vi "Asylum_Driver_GetXYSetPoints.vi"(8 "error in (no error)":errorcluster, 11 "Application":refnum<k7>) -> (0 "error out":errorcluster, 1 "Y PIS Controls":T1, 2 "X PIS Controls":T1, 3 "Application":refnum<k7>)   [LabVIEW 2019]
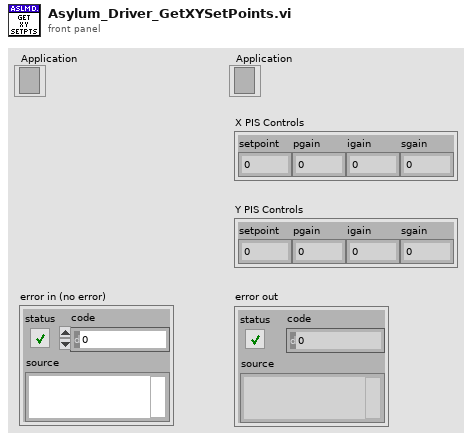
[diagram p1: front panel]
types:
  T1 = cluster{"setpoint":dbl, "pgain":dbl, "igain":dbl, "sgain":dbl}
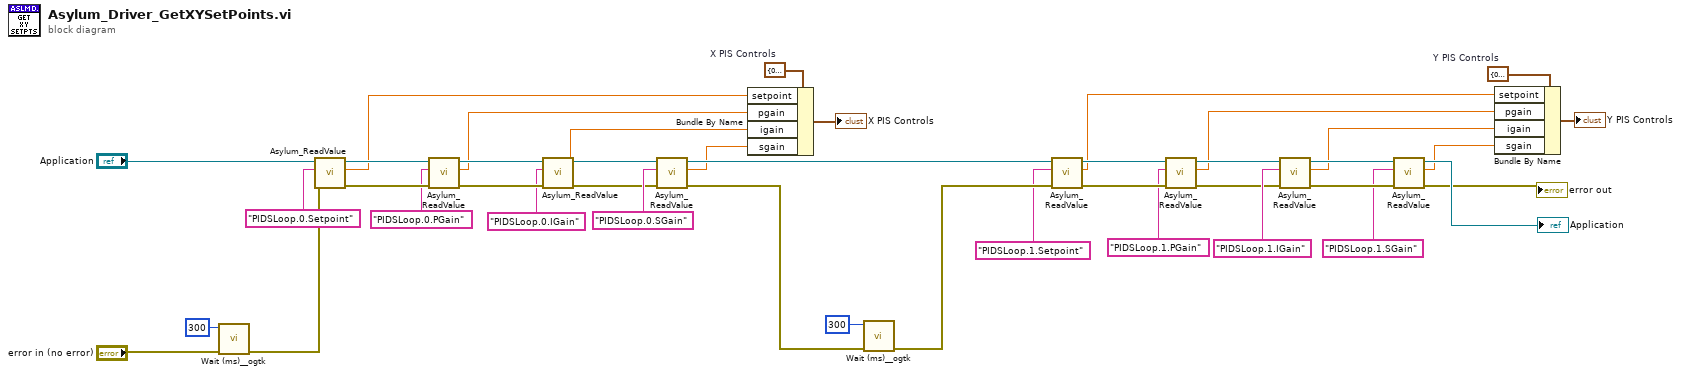
[diagram p0: block diagram]
diagram:
  w25 = T1 {"setpoint"=0.0, "pgain"=0.0, "igain"=0.0, "sgain"=0.0}  # Y PIS Controls
  w37 = T1 {"setpoint"=0.0, "pgain"=0.0, "igain"=0.0, "sgain"=0.0}  # X PIS Controls
  n1 = call <userlib>:"Wait (ms)__ogtk.vi"("error in (no error)"="error in (no error)", "milliseconds to wait"=u32 300) -> ("error out"=w41:errorcluster)  [unwired: 8 in, 1 out]
  n2 = call <userlib>:"Asylum_ReadValue.vi"("error in (no error)"=w41, "Value"="PIDSLoop.0.Setpoint", "Application"="Application") -> ("error out"=w28:errorcluster, "Value"=w29:dbl, "Application"=w36:refnum<k7>)  [unwired: 6 in]
  n3 = call <userlib>:"Asylum_ReadValue.vi"("error in (no error)"=w28, "Value"="PIDSLoop.0.PGain", "Application"=w36) -> ("error out"=w27:errorcluster, "Value"=w30:dbl, "Application"=w35:refnum<k7>)  [unwired: 6 in]
  n4 = call <userlib>:"Asylum_ReadValue.vi"("error in (no error)"=w27, "Value"="PIDSLoop.0.IGain", "Application"=w35) -> ("error out"=w26:errorcluster, "Value"=w34:dbl, "Application"=w33:refnum<k7>)  [unwired: 6 in]
  n5 = call <userlib>:"Asylum_ReadValue.vi"("error in (no error)"=w26, "Value"="PIDSLoop.0.SGain", "Application"=w33) -> ("error out"=w10:errorcluster, "Value"=w1:dbl, "Application"=w17:refnum<k7>)  [unwired: 6 in]
  n6 = Bundle By Name(cluster=w37, "setpoint"=w29, "pgain"=w30, "igain"=w34, "sgain"=w1) -> (→"X PIS Controls":T1)
  n7 = call <userlib>:"Wait (ms)__ogtk.vi"("error in (no error)"=w10, "milliseconds to wait"=u32 300) -> ("error out"=w9:errorcluster)  [unwired: 8 in, 1 out]
  n8 = call <userlib>:"Asylum_ReadValue.vi"("error in (no error)"=w9, "Value"="PIDSLoop.1.Setpoint", "Application"=w17) -> ("error out"=w21:errorcluster, "Value"=w16:dbl, "Application"=w18:refnum<k7>)  [unwired: 6 in]
  n9 = call <userlib>:"Asylum_ReadValue.vi"("error in (no error)"=w21, "Value"="PIDSLoop.1.PGain", "Application"=w18) -> ("error out"=w22:errorcluster, "Value"=w8:dbl, "Application"=w19:refnum<k7>)  [unwired: 6 in]
  n10 = call <userlib>:"Asylum_ReadValue.vi"("error in (no error)"=w22, "Value"="PIDSLoop.1.IGain", "Application"=w19) -> ("error out"=w23:errorcluster, "Value"=w14:dbl, "Application"=w20:refnum<k7>)  [unwired: 6 in]
  n11 = call <userlib>:"Asylum_ReadValue.vi"("error in (no error)"=w23, "Value"="PIDSLoop.1.SGain", "Application"=w20) -> ("error out"=→"error out":errorcluster, "Value"=w13:dbl, "Application"=→"Application":refnum<k7>)  [unwired: 6 in]
  n12 = Bundle By Name(cluster=w25, "setpoint"=w16, "pgain"=w8, "igain"=w14, "sgain"=w13) -> (→"Y PIS Controls":T1)
